vi "test-unscented-kalman-filter-1.vi"() -> (3 "Test good":bool)   [LabVIEW 2019]
uses:
  <vilib>/Analysis/Matrix/Datatypes/RealMatrix.ctl
  <vilib>/Rock Robotics/WPI/ThirdParty/JAS_Junk/TrajLib/TRAJ_STATE.ctl
  <vilib>/Rock Robotics/WPI/ThirdParty/JAS_Junk/TrajLib/POSE2D.ctl
  <vilib>/Rock Robotics/WPI/ThirdParty/JAS_Junk/TrajLib/TRANSLATION2D.ctl
  <vilib>/Rock Robotics/WPI/ThirdParty/JAS_Junk/TrajLib/ROTATION2D.ctl
  <vilib>/Rock Robotics/WPI/ThirdParty/JAS_Junk/TrajLib/MatrixHelper_CoerceSize.vi
  <vilib>/Rock Robotics/WPI/ThirdParty/JAS_Junk/TrajLib/Rotation_CreateAngle.vi
  <vilib>/Rock Robotics/WPI/ThirdParty/JAS_Junk/TrajLib/Translation_Create.vi
  <vilib>/Analysis/1siggen.llb/Gaussian White Noise.vi
  <vilib>/Analysis/Matrix/Numeric/Add/Add - RM,RM.vi
  <vilib>/Analysis/Matrix/Numeric/Subtract/Subtract - RM,RM.vi
  <vilib>/Analysis/7linalg.llb/Solve Linear Equations (multiple right hand).vi
  <vilib>/Rock Robotics/WPI/ThirdParty/JAS_Junk/TrajLib/CallbackHelp_MatrixPlus.vi
  <vilib>/Rock Robotics/WPI/ThirdParty/JAS_Junk/TrajLib/CallbackHelp_MatrixMinus.vi
  <vilib>/Rock Robotics/WPI/ThirdParty/JAS_Junk/TrajLib/Trajectory_Library.lvlib
  <vilib>/Analysis/Matrix/NI_Matrix.lvlib
  <vilib>/Analysis/NI_AALPro.lvlib
panel:
  out "Traj sample":T1={"TimeSeconds"=0.0, "Velocity"=0.0, "Acceleration"=0.0, "POSE"={"TRANSLATION"={"X"=0.0, "Y"=0.0}, "ROTATION"={"VALUE"=0.0, "COS"=1.0, "SIN"=0.0}}, "Curvature"=0.0} {"POSE"."ROTATION"."SIN" format="%13.4f"; "POSE"."ROTATION"."COS" format="%13.4f"; "POSE"."ROTATION"."VALUE" format="%13.4f"; "POSE"."TRANSLATION"."Y" format="%14.3f"; "POSE"."TRANSLATION"."X" format="%14.3f"}
  out "Error 14":bool
  out "xHat":T5
  out "OutputTRAJ_STATE":T1={"TimeSeconds"=0.0, "Velocity"=0.0, "Acceleration"=0.0, "POSE"={"TRANSLATION"={"X"=0.0, "Y"=0.0}, "ROTATION"={"VALUE"=0.0, "COS"=1.0, "SIN"=0.0}}, "Curvature"=0.0} {"POSE"."ROTATION"."SIN" format="%13.4f"; "POSE"."ROTATION"."COS" format="%13.4f"; "POSE"."ROTATION"."VALUE" format="%13.4f"; "POSE"."TRANSLATION"."Y" format="%14.3f"; "POSE"."TRANSLATION"."X" format="%14.3f"}
  out "Error 13":bool
  out "Sze Coerced":bool
  out "Error 12":errorcluster
  out "Return 2":T5
  out "Error 11":bool
  out "Error 10":bool
  out "Error 8":bool
  out "error":i32
  out "Solution Matrix":T5
  out "Get Dynam":T5
  out "Error 9":bool
  out "Size Coerced":bool
  out "TrueXHat":T5
  out "Error 3":bool
  out "Error 2":bool
  out "Error":bool
  out "r":T5
  out "SizeCoerced":bool
  out "X":T5
  out "Error 7":bool
  out "B":T5
  out "Y 2":T5
  out "Error 6":bool
  out "Error 5":bool
  out "Error 00":errorcluster
  # "assertEquals(finalPosition.poseMeters.getTranslation().getX(), observer.getXhat(0), 0.25);\n    assertEquals(finalPosition.poseMeters.getTranslation().getY(), observer.getXhat(1), 0.25);\n    assertEquals(finalPosition.poseMeters.getRotation().getRadians(), observer.getXhat(2), 1.0);\n    assertEquals(0.0, observer.getXhat(3), 1.0);\n    assertEquals(0.0, observer.getXhat(4), 1.0);"
  # "24.7"
  # "19.68"
  # "-.4372"
  # "0"
  # "0"
  # "Traj end\n          24.73, \n         19.68, \n          Degrees(5.846)"
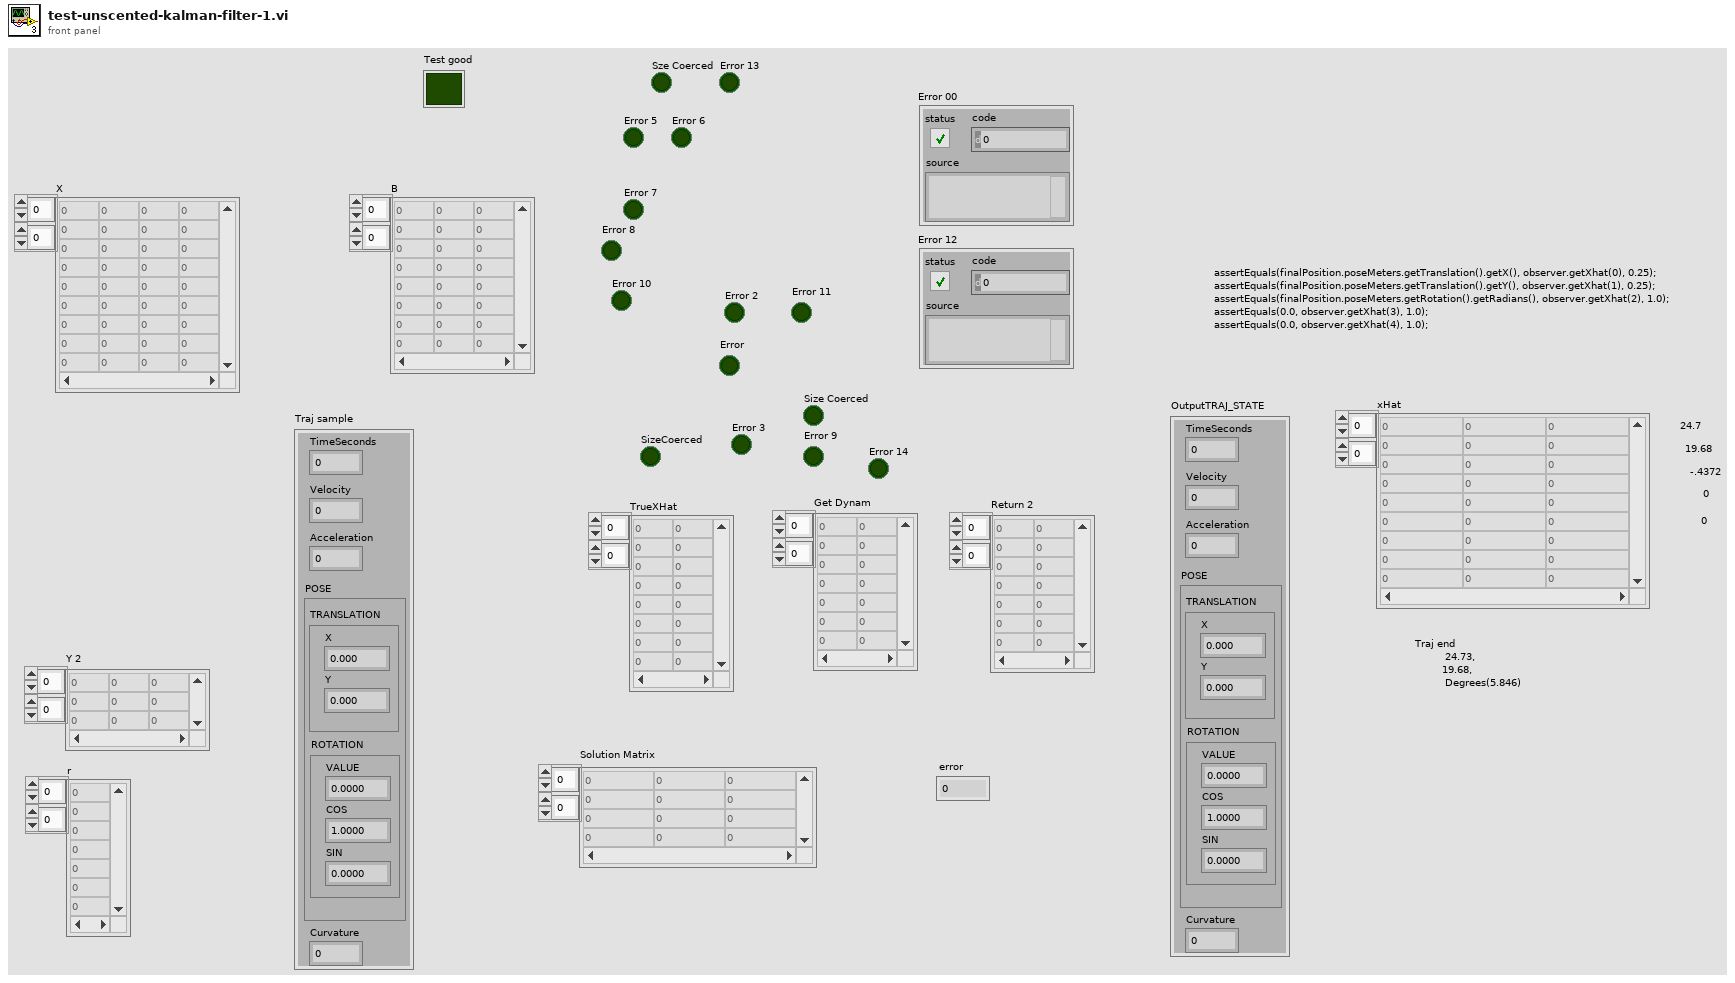
[diagram p1: front panel]
types:
  T1 = typedef "Trajectory_Library.lvlib/TRAJ_STATE.ctl" = cluster{"TimeSeconds":dbl, "Velocity":dbl, "Acceleration":dbl, "POSE":T2, "Curvature":dbl}
  T2 = typedef "Trajectory_Library.lvlib/POSE2D.ctl" = cluster{"TRANSLATION":T3, "ROTATION":T4}
  T3 = typedef "Trajectory_Library.lvlib/TRANSLATION2D.ctl" = cluster{"X":dbl, "Y":dbl}
  T4 = typedef "Trajectory_Library.lvlib/ROTATION2D.ctl" = cluster{"VALUE":dbl, "COS":dbl, "SIN":dbl}
  T5 = typedef "NI_Matrix.lvlib/RealMatrix.ctl" = dbl[][]
  T6 = typedef "Trajectory_Library.lvlib/TRAJ_CONFIG.ctl" = cluster{"MaxVelocity":dbl, "Max Acceleration":dbl, "StartVelocity":dbl, "End Velocity":dbl, "Reversed":bool, "DiffDrKineConstntDefined":bool, "CentAcellConstntDefined":bool, "DiffDrVoltConstntDefined":bool, "DIFF_DRIVE_KINE_CONSTRAINT":T7, "CENTRIPETAL_ACCEL_CONSTRAINT":T9, "SwerveDrKineConstntDefined":bool, "SWERVE_DRIVE_KINE_CONSTRAINT":T10, "DIFF_DRIVE_VOLTAGE_CONSTRAINT":T12, "MECANUM_DRIVE_KINE_CONSTRAINT":T14, "MecanumDrKineConstntDefined":bool}
  T7 = typedef "Trajectory_Library.lvlib/TRAJ_CONSTRAINT_DIIF_DRIVE_KINEMATICS.ctl" = cluster{"Max Speed (M/S)":dbl, "DIFF_DRIVE_KINEMATICS":T8, "Max Accel (M/S2)":dbl}
  T8 = typedef "Trajectory_Library.lvlib/DIFF_DRIVE_KINEMATICS.ctl" = cluster{"TrackWidth_Meters":dbl}
  T9 = typedef "Trajectory_Library.lvlib/TRAJ_CONSTRAINT_CENTRIPETAL_ACCEL.ctl" = cluster{"Max Cent Accel":dbl}
  T10 = typedef "Trajectory_Library.lvlib/TRAJ_CONSTRAINT_SWERVE_DRIVE_KINEMATICS.ctl" = cluster{"Max Speed (M/S)":dbl, "SwerveKinematics":T11}
  T11 = typedef "Trajectory_Library.lvlib/SWERVE_DRIVE_KINEMATICS.ctl" = cluster{"NumModules":i32, "InverseKinematics":T5, "ForwardKinematics":T5, "Modules":T3[], "PrevCoR":T3}
  T12 = typedef "Trajectory_Library.lvlib/TRAJ_CONSTRAINT_DIIF_DRIVE_VOLTAGE.ctl" = cluster{"Max Voltage":dbl, "DIFF_DRIVE_KINEMATICS":T8, "SIMPLE_MOTOR_FF":T13}
  T13 = typedef "Trajectory_Library.lvlib/SIMPLE_MOTOR_FF.ctl" = cluster{"Ks":dbl, "Kv":dbl, "Ka":dbl}
  T14 = typedef "Trajectory_Library.lvlib/TRAJ_CONSTRAINT_MECA_DRIVE_KINEMATICS.ctl" = cluster{"Max Speed (M/S)":dbl, "MECA_DRIVE_KINEMATICS":T15}
  T15 = typedef "Trajectory_Library.lvlib/MECA_DRIVE_KINEMATICS.ctl" = cluster{"FrontLeft":T3, "FrontRight":T3, "RearLeft":T3, "RearRight":T3, "InverseKinematics":T5, "ForwardKinematics":T5, "PrevCoR":T3}
  T16 = typedef "Trajectory_Library.lvlib/TRAJECTORY.ctl" = cluster{"TotalTImeSecs":dbl, "States":T1[]}
  T17 = typedef "Trajectory_Library.lvlib/UNSCENTED_KALMAN_FILTER.ctl" = cluster{"m_P":T5, "m_xHat":T5, "States":i32, "Outputs":i32, "m_ContR":T5, "m_ContQ":T5, "m_SigmasF":T5, "m_dT_Sec":dbl, "MERWE_SCALED_SIGMA_PTS":T18, "meanFuncX":T19, "meanFuncY":T19, "residualFuncX":T19, "residualFuncY":T19, "addFuncX":T19, "addFuncXExtra":variant, "residualFuncYExtra":variant, "residualFuncXExtra":variant, "MeanFuncYExtra":variant, "MeanFuncXExtra":variant, "Inputs":i32}
  T18 = typedef "Trajectory_Library.lvlib/MERWE_SCALED_SIGMA_PTS.ctl" = cluster{"m_Wm":T5, "States":i32, "Alpha":dbl, "m_Wc":T5, "Kappa":i32}
  T19 = typedef "Trajectory_Library.lvlib/CALLBACK_FUNC_TYPE.ctl" = refnum<vi>
  T20 = typedef "Trajectory_Library.lvlib/UNSCENTED_KALMAN_CORRECT_FUNC_GROUP.ctl" = cluster{"H_Func":T19, "meanFuncY":T19, "residualFuncY":T19, "residualFuncX":T19, "addFuncX":T19, "H_FuncExtra":variant, "MeanFuncYExtra":variant, "residualFuncYExtra":variant, "residualFuncXExtra":variant, "addFuncXExtra":variant}
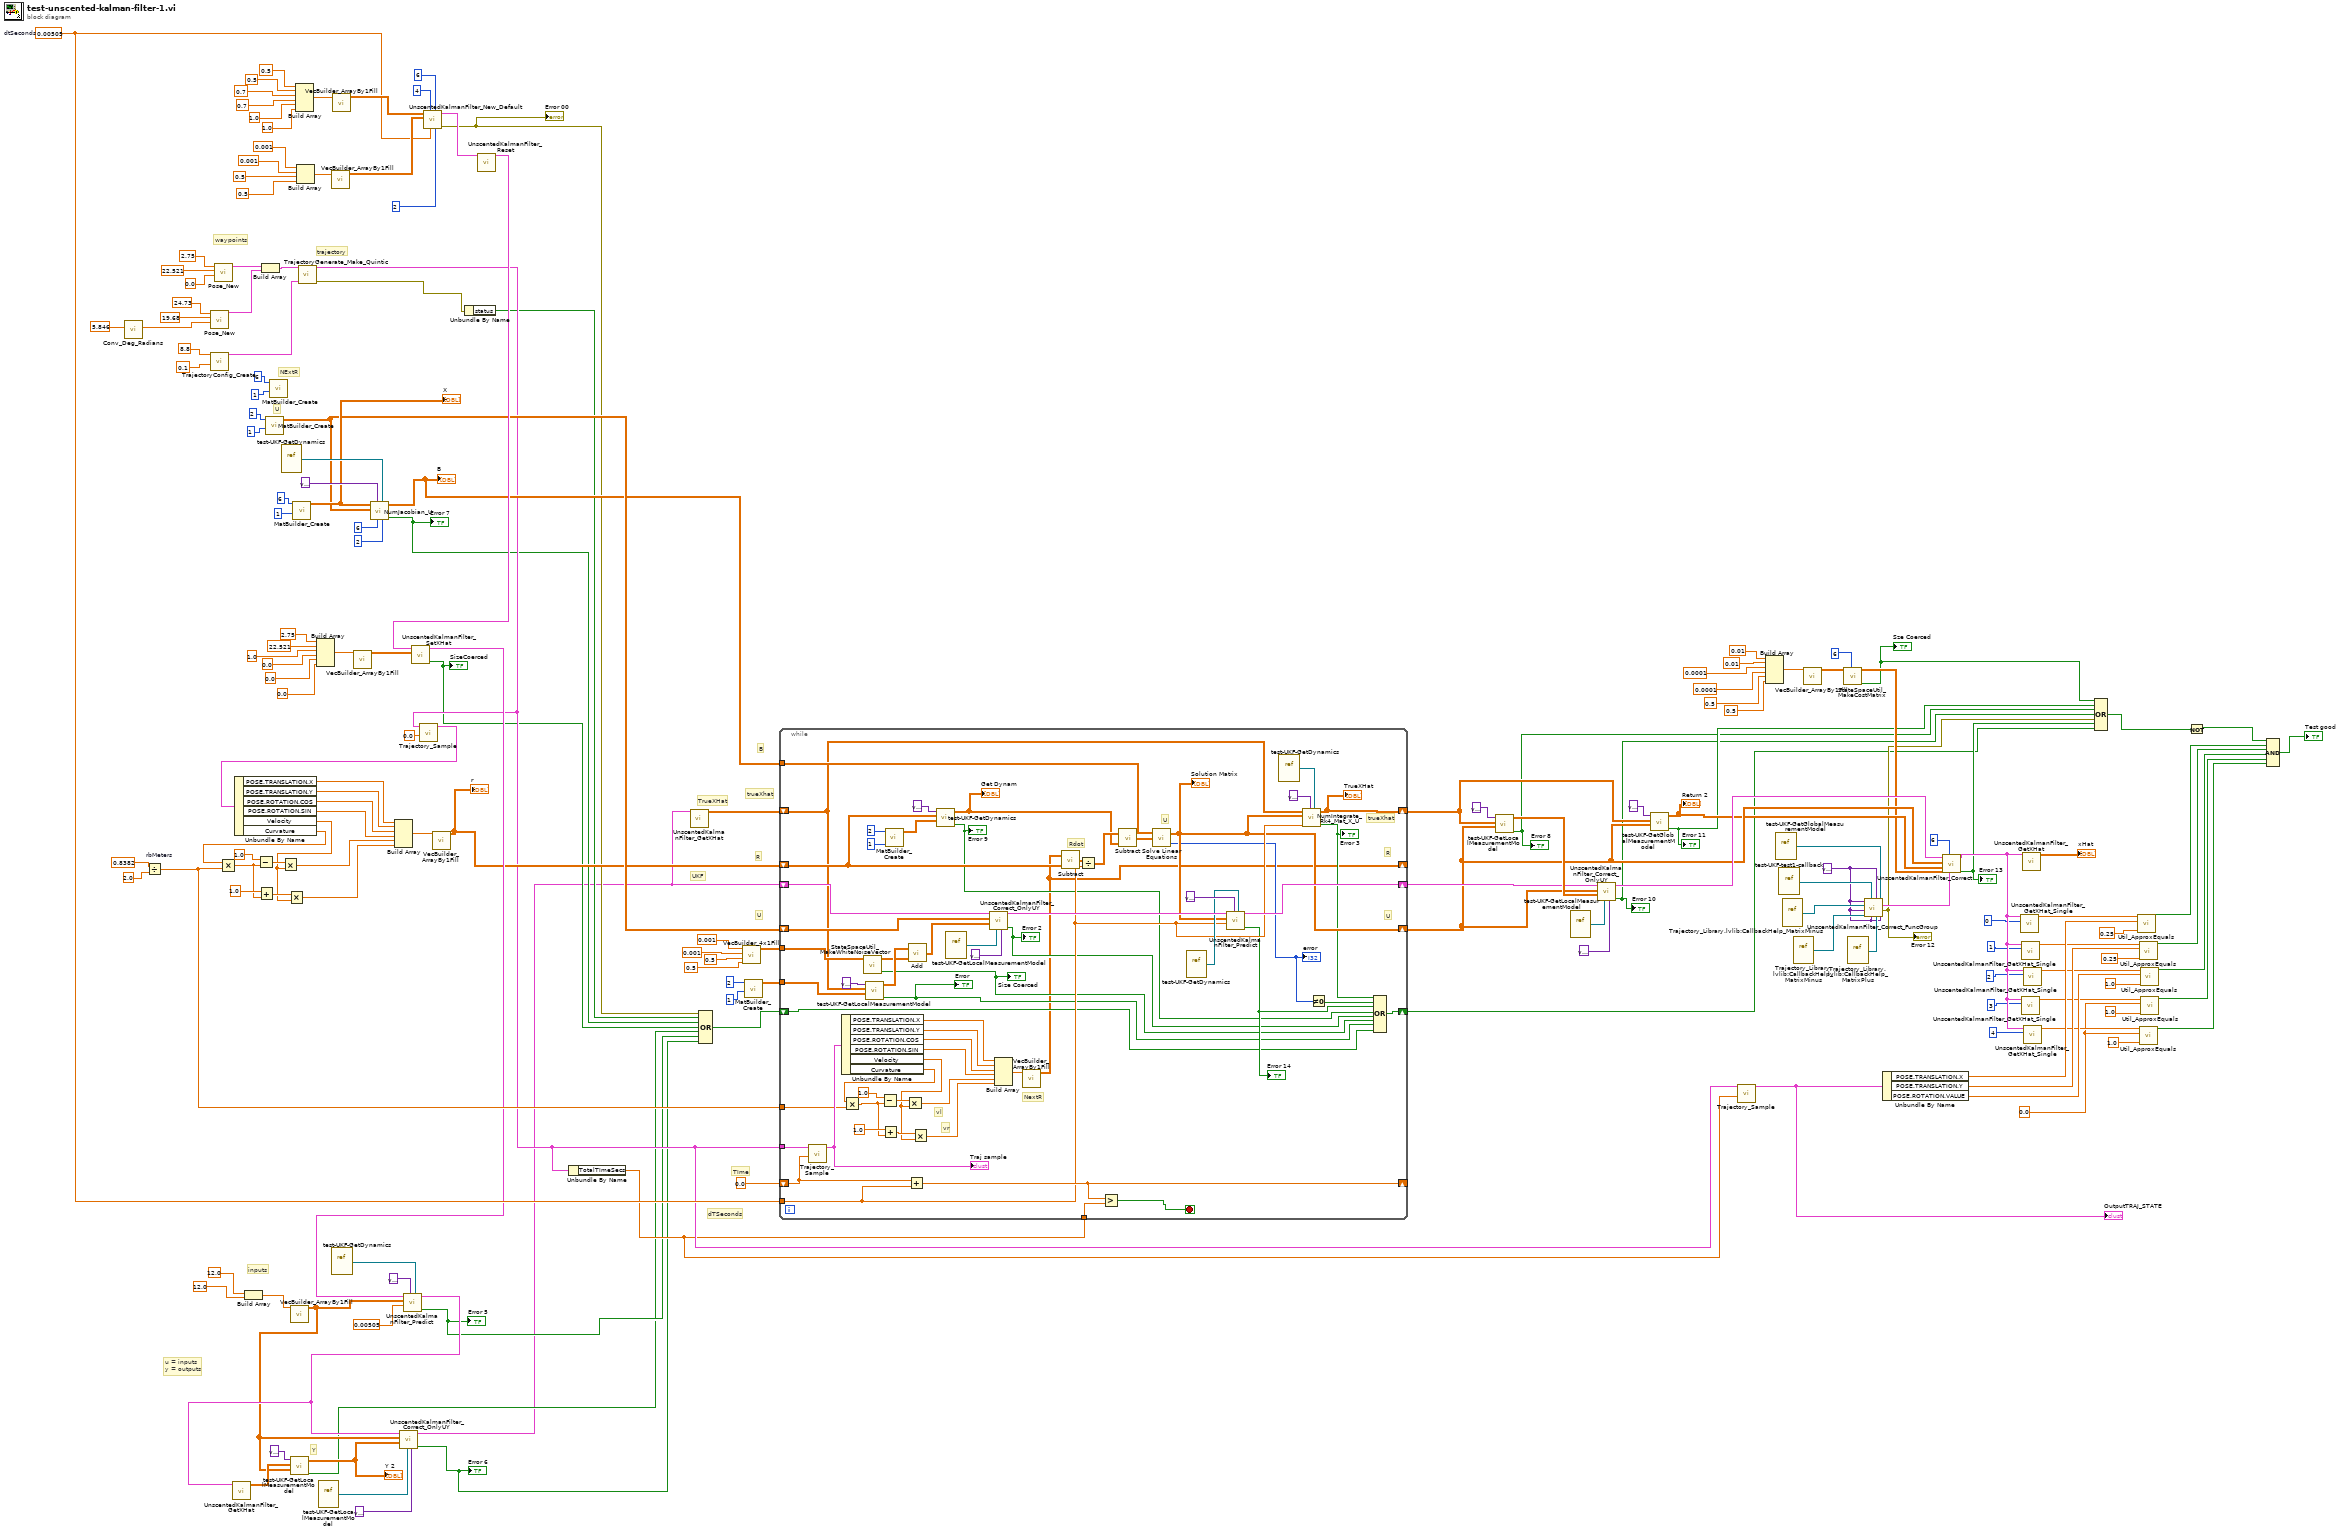
[diagram p0: block diagram]
diagram:
  w32 = 0.0 ("Value 2")
  w56 = variant ("H_FuncExtra")
  w93 = 0.00505  # dtSeconds
  # "UKF"
  # "B"
  # "trueXhat"
  # "dTSeconds"
  # "R"
  # "U"
  # "TrueXHat"
  # "TIme"
  # "U"
  # "NExtR"
  # "trajectory"
  # "waypoints"
  # "u = inputs\ny = outputs"
  # "inputs"
  # "Y"
  n1 = call <vilib>:"Conv_Deg_Radians.vi"("Degress"=5.846 ("Heading")) -> ("Radians"=w46:dbl)  [unwired: 10 in]
  n2 = Divide "rbMeters"(x=0.8382, y=2.0) -> (x/y=w92:dbl)
  n3 = call <vilib>:"Pose_New.vi"("Heading"=w46, "Y"=19.68, "X"=24.73) -> ("out POSe"=w135:T2)  [unwired: 8 in]
  n4 = call <vilib>:"TrajectoryConfig_Create.vi"("MaxAcceleration"=0.1, "MaxVelocity"=8.8) -> ("TRAJECTORY_CONFIG"=w131:T6)  [unwired: 9 in]
  n5 = call <vilib>:"Pose_New.vi"("Heading"=0.0, "Y"=22.521, "X"=2.75) -> ("out POSe"=w136:T2)  [unwired: 8 in]
  n6 = Build Array(12.0 ("element"), 12.0 ("element")) -> (w154:dbl[])
  n7 = Build Array(w136, w135) -> (w132:T2[])
  n8 = call <vilib>:"MatBuilder_Create.vi"("Columns"=1, "Rows"=2) -> ("output matrix"=w81:T5)  [unwired: 9 in]
  n9 = call <vilib>:"MatBuilder_Create.vi"("Columns"=1, "Rows"=6) -> ()  [unwired: 9 in, 1 out]
  n10 = vi-ref "test-UKF-GetDynamics.vi"() -> (w122:refnum<vi>)
  n11 = call <vilib>:"VecBuilder_ArrayBy1Fill.vi"("R Array"=w154) -> ("Output Vector"=w145:T5)  [unwired: 10 in]
  n12 = call <vilib>:"MatBuilder_Create.vi"("Columns"=1, "Rows"=6) -> ("output matrix"=w120:T5)  [unwired: 9 in]
  "X" <- w120
  n13 = Build Array(0.5 ("element"), 0.5 ("element"), 0.7 ("element"), 0.7 ("element"), 1.0 ("element"), 1.0 ("element")) -> (w172:dbl[])
  n14 = Build Array(0.001 ("element"), 0.001 ("element"), 0.5 ("element"), 0.5 ("element")) -> (w161:dbl[])
  n15 = call <vilib>:"TrajectoryGenerate_Make_Quintic.vi"("traj_config"=w131, "waypointPOSE"=w132) -> ("error out"=w10:errorcluster, "TRAJECTORY"=w50:T16)  [unwired: 8 in]
  n16 = Build Array(2.75 ("element"), 22.521 ("element"), 1.0 ("element"), 0.0 ("element"), 0.0 ("element"), 0.0 ("element")) -> (w112:dbl[])
  n17 = vi-ref "test-UKF-GetLocalMeasurementModel.vi"() -> (w149:refnum<vi>)
  n18 = call <vilib>:"VecBuilder_ArrayBy1Fill.vi"("R Array"=w161) -> ("Output Vector"=w160:T5)  [unwired: 10 in]
  n19 = vi-ref "test-UKF-GetDynamics.vi"() -> (w151:refnum<vi>)
  n20 = call <vilib>:"VecBuilder_ArrayBy1Fill.vi"("R Array"=w172) -> ("Output Vector"=w159:T5)  [unwired: 10 in]
  n21 = call <vilib>:"VecBuilder_ArrayBy1Fill.vi"("R Array"=w112) -> ("Output Vector"=w111:T5)  [unwired: 10 in]
  n22 = call <vilib>:"NumJacobian_U.vi"("Inputs"=2, "F_FUNC"=w122, "Rows"=6, "ExtraPassedData"=variant ("F_Func_ExtraData"), "U"=w81, "X"=w120) -> ("Error"=w11:bool, "Result"=w79:T5)  [unwired: 4 in]
  "B" <- w79
  "Error 7" <- w11
  n23 = call <vilib>:"Trajectory_Sample.vi"("Time"=0.0, "InputTRAJECTORY"=w50) -> ("OutputTRAJ_STATE"=w109:T1)  [unwired: 9 in]
  n24 = Unbundle By Name(w109) -> ("POSE.TRANSLATION.X"=w108:dbl, "POSE.TRANSLATION.Y"=w107:dbl, "POSE.ROTATION.COS"=w106:dbl, "POSE.ROTATION.SIN"=w105:dbl, "Velocity"=w98:dbl, "Curvature"=w104:dbl)
  n25 = Multiply(x=w104, y=w92) -> (x*y=w101:dbl)
  n26 = Subtract(x=1.0, y=w101) -> (x-y=w99:dbl)
  n27 = Add(x=1.0, y=w101) -> (x+y=w100:dbl)
  n28 = Multiply(x=w99, y=w98) -> (x*y=w97:dbl)
  n29 = Multiply(x=w100, y=w98) -> (x*y=w96:dbl)
  n30 = Build Array(w108, w107, w106, w105, w97, w96) -> (w95:dbl[])
  n31 = call <vilib>:"UnscentedKalmanFilter_New_Default.vi"("Inputs"=2, "States"=6, "dt_Seconds"=w93, "Outputs"=4, "MeasurementStdDevs"=w160, "StateStdDevs"=w159) -> ("Error"=w8:errorcluster, "UnscentedKalmanFiilter"=w157:T17)  [unwired: 4 in]
  "Error 00" <- w8
  n32 = call <vilib>:"VecBuilder_ArrayBy1Fill.vi"("R Array"=w95) -> ("Output Vector"=w80:T5)  [unwired: 10 in]
  "r" <- w80
  n33 = Unbundle By Name(w10) -> ("status"=w9:bool)
  n34 = call <vilib>:"UnscentedKalmanFilter_Reset.vi"("in UnscentedKalmanFiilter"=w157) -> ("out UnscentedKalmanFiilter"=w119:T17)  [unwired: 10 in]
  n35 = call <vilib>:"UnscentedKalmanFilter_SetXHat.vi"("xHat"=w111, "in UnscentedKalmanFiilter"=w119) -> ("SizeCoerced"=w13:bool, "out UnscentedKalmanFiilter"=w83:T17)  [unwired: 8 in]
  "SizeCoerced" <- w13
  n36 = call <vilib>:"UnscentedKalmanFilter_Predict.vi"("f_Func"=w151, "F_Func_ExtraData"=variant, "dT_Seconds"=0.00505, "U"=w145, "in UnscentedKalmanFiilter"=w83) -> ("Error"=w16:bool, "out UnscentedKalmanFiilter"=w148:T17)  [unwired: 5 in]
  "Error 5" <- w16
  n37 = call <vilib>:"UnscentedKalmanFilter_GetXHat.vi"("in UnscentedKalmanFiilter"=w148) -> ("xHat"=w146:T5)  [unwired: 10 in]
  n38 = call "test-UKF-GetLocalMeasurementModel.vi"("U"=w145, "X"=w146, "Variant"=variant) -> ("Error"=w14:bool, "Return"=w144:T5)  [unwired: 7 in]
  "Y 2" <- w144
  n39 = call <vilib>:"UnscentedKalmanFilter_Correct_OnlyUY.vi"("H_ExtraData"=variant ("F_Func_ExtraData"), "H_Func"=w149, "Y"=w144, "U"=w145, "in UnscentedKalmanFiilter"=w148) -> ("Error"=w15:bool, "out UnscentedKalmanFiilter"=w1:T17)  [unwired: 5 in]
  "Error 6" <- w15
  n40 = Unbundle By Name(w50) -> ("TotalTImeSecs"=w49:dbl)
  n41 = call <vilib>:"UnscentedKalmanFilter_GetXHat.vi"("in UnscentedKalmanFiilter"=w1) -> ("xHat"=w91:T5)  [unwired: 10 in]
  n42 = Compound Arithmetic op=OR(w8, w9, w11, w13, w14, w16, w15) -> (w12:bool)
  n43 = call <vilib>:"VecBuilder_4x1Fill.vi"("R3"=0.5, "R2"=0.5, "R1"=0.001, "R0"=0.001) -> ("output matrix"=w82:T5)  [unwired: 7 in]
  n44 = call <vilib>:"MatBuilder_Create.vi"("Columns"=1, "Rows"=2) -> ("output matrix"=w88:T5)  [unwired: 9 in]
  n45 = while {
    shift-right: [w235] -> _
    shift-left: 0.0 -> [w237]
    tunnel: w93 -> [w190]
    tunnel: w50 -> [w234]
    tunnel: w49 -> [w233]
    tunnel: w92 -> [w218]
    tunnel: w88 -> [w216]
    shift-right: [w197] -> w76
    shift-left: w1 -> [w215]
    tunnel: w82 -> [w214]
    shift-right: [w188] -> w53
    shift-left: w81 -> [w208]
    shift-right: [w176] -> _
    shift-left: w80 -> [w204]
    tunnel: w79 -> [w198]
    shift-right: [w189] -> w72
    shift-left: w91 -> [w191]
    shift-right: [w180] -> w7
    shift-left: w12 -> [w177]
    stop <- w236 stop-if-true
    # "vr"
    # "vl"
    # "Rdot"
    # "trueXhat"
    # "R"
    # "U"
    # "U"
    # "NextR"
    n46 = call <vilib>:"Trajectory_Sample.vi"("Time"=w237, "InputTRAJECTORY"=w234) -> ("OutputTRAJ_STATE"=w219:T1)  [unwired: 9 in]
    "Traj sample" <- w219
    n47 = Unbundle By Name(w219) -> ("POSE.TRANSLATION.X"=w232:dbl, "POSE.TRANSLATION.Y"=w231:dbl, "POSE.ROTATION.COS"=w230:dbl, "POSE.ROTATION.SIN"=w229:dbl, "Velocity"=w222:dbl, "Curvature"=w228:dbl)
    n48 = Multiply(x=w228, y=w218) -> (x*y=w225:dbl)
    n49 = call <vilib>:"StateSpaceUtil_MakeWhiteNoiseVector.vi"("StdDevs"=w214) -> ("Size Coerced"=w179:bool, "WhiteNoise"=w211:T5)  [unwired: 9 in]
    "Size Coerced" <- w179
    n50 = call "test-UKF-GetLocalMeasurementModel.vi"("U"=w216, "X"=w191, "Variant"=variant) -> ("Error"=w178:bool, "Return"=w212:T5)  [unwired: 7 in]
    "Error" <- w178
    n51 = Subtract(x=1.0, y=w225) -> (x-y=w223:dbl)
    n52 = Add(x=1.0, y=w225) -> (x+y=w224:dbl)
    n53 = call <vilib>:"MatBuilder_Create.vi"("Columns"=1, "Rows"=2) -> ("output matrix"=w200:T5)  [unwired: 9 in]
    n54 = Multiply(x=w223, y=w222) -> (x*y=w221:dbl)
    n55 = Add(x=w237, y=w190) -> (x+y=w235:dbl)
    n56 = call-poly <vilib>:"Add.vi"("Real Matrix B"=w211, "Real Matrix A"=w212) -> ("A + B"=w213:T5)
    n57 = Multiply(x=w224, y=w222) -> (x*y=w220:dbl)
    n58 = call "test-UKF-GetDynamics.vi"("U"=w200, "X"=w204, "Variant"=variant) -> ("Error"=w182:bool, "Return"=w183:T5)  [unwired: 7 in]
    "Error 9" <- w182
    "Get Dynam" <- w183
    n59 = vi-ref "test-UKF-GetLocalMeasurementModel.vi"() -> (w210:refnum<vi>)
    n60 = call <vilib>:"UnscentedKalmanFilter_Correct_OnlyUY.vi"("H_ExtraData"=variant, "H_Func"=w210, "Y"=w213, "U"=w208, "in UnscentedKalmanFiilter"=w215) -> ("Error"=w181:bool, "out UnscentedKalmanFiilter"=w196:T17)  [unwired: 5 in]
    "Error 2" <- w181
    n61 = Build Array(w232, w231, w230, w229, w221, w220) -> (w207:dbl[])
    n62 = call <vilib>:"VecBuilder_ArrayBy1Fill.vi"("R Array"=w207) -> ("Output Vector"=w176:T5)  [unwired: 10 in]
    n63 = call-poly <vilib>:"Subtract.vi"("Real Matrix B"=w204, "Real Matrix A"=w176) -> ("A - B"=w206:T5)
    n64 = Divide(x=w206, y=w190) -> (x/y=w205:T5)
    n65 = Greater?(x=w235, y=w233) -> (0:w236:bool)
    n66 = call-poly <vilib>:"Subtract.vi"("Real Matrix B"=w183, "Real Matrix A"=w205) -> ("A - B"=w199:T5)
    n67 = call-poly <vilib>:"Solve Linear Equations.vi"("Known Matrix"=w199, "Input Matrix"=w198) -> ("error"=w185:i32, "Solution Matrix"=w188:T5)  [unwired: 1 in]
    "Solution Matrix" <- w188
    "error" <- w185
    n68 = vi-ref "test-UKF-GetDynamics.vi"() -> (w194:refnum<vi>)
    n69 = call <vilib>:"UnscentedKalmanFilter_Predict.vi"("f_Func"=w194, "F_Func_ExtraData"=variant, "dT_Seconds"=w190, "U"=w188, "in UnscentedKalmanFiilter"=w196) -> ("Error"=w184:bool, "out UnscentedKalmanFiilter"=w197:T17)  [unwired: 5 in]
    "Error 14" <- w184
    n70 = vi-ref "test-UKF-GetDynamics.vi"() -> (w192:refnum<vi>)
    n71 = call <vilib>:"NumIntegrate_Rk4_Mat_X_U.vi"("Func_X_U_Extra"=w192, "PassedData"=variant, "dT_Seconds"=w190, "U"=w188, "X"=w191) -> ("Error"=w187:bool, "OUTPUT"=w189:T5)  [unwired: 5 in]
    "Error 3" <- w187
    "TrueXHat" <- w189
    n72 = Not Equal To 0?(x=w185) -> (x != 0?=w186:bool)
    n73 = Compound Arithmetic op=OR(w187, w186, w184, w182, w181, w179, w178, w177) -> (w180:bool)
  }
  n74 = call "test-UKF-GetLocalMeasurementModel.vi"("U"=w53, "X"=w72, "Variant"=variant) -> ("Error"=w27:bool, "Return"=w77:T5)  [unwired: 7 in]
  "Error 8" <- w27
  n75 = vi-ref "test-UKF-GetLocalMeasurementModel.vi"() -> (w75:refnum<vi>)
  n76 = call <vilib>:"UnscentedKalmanFilter_Correct_OnlyUY.vi"("H_ExtraData"=variant, "H_Func"=w75, "Y"=w77, "U"=w53, "in UnscentedKalmanFiilter"=w76) -> ("Error"=w26:bool, "out UnscentedKalmanFiilter"=w55:T17)  [unwired: 5 in]
  "Error 10" <- w26
  n77 = call "test-UKF-GetGlobalMeasurementModel.vi"("U"=w53, "X"=w72, "Variant"=variant) -> ("Error"=w28:bool, "Return"=w52:T5)  [unwired: 7 in]
  "Error 11" <- w28
  "Return 2" <- w52
  n78 = call <vilib>:"Trajectory_Sample.vi"("Time"=w49, "InputTRAJECTORY"=w50) -> ("OutputTRAJ_STATE"=w45:T1)  [unwired: 9 in]
  "OutputTRAJ_STATE" <- w45
  n79 = Build Array(0.01 ("element"), 0.01 ("element"), 0.0001 ("element"), 0.0001 ("element"), 0.5 ("element"), 0.5 ("element")) -> (w63:dbl[])
  n80 = vi-ref "test-UKF-GetGlobalMeasurementModel.vi"() -> (w57:refnum<vi>)
  n81 = vi-ref "test-UKF-test1-callback.vi"() -> (w58:refnum<vi>)
  n82 = vi-ref "Trajectory_Library.lvlib:CallbackHelp_MatrixMinus.vi"() -> (w59:refnum<vi>)
  n83 = vi-ref "Trajectory_Library.lvlib:CallbackHelp_MatrixMinus.vi"() -> (w60:refnum<vi>)
  n84 = call <vilib>:"VecBuilder_ArrayBy1Fill.vi"("R Array"=w63) -> ("Output Vector"=w64:T5)  [unwired: 10 in]
  n85 = call <vilib>:"StateSpaceUtil_MakeCostMatrix.vi"("States"=6, "Costs"=w64) -> ("Sze Coerced"=w29:bool, "Costs Matrix"=w51:T5)  [unwired: 8 in]
  "Sze Coerced" <- w29
  n86 = vi-ref "Trajectory_Library.lvlib:CallbackHelp_MatrixPlus.vi"() -> (w61:refnum<vi>)
  n87 = call <vilib>:"UnscentedKalmanFilter_Correct_FuncGroup.vi"("addFuncXExtra"=w56, "H_Func"=w57, "AddFuncX"=w61, "H_FuncExtra"=w56, "residualFuncXExtra"=w56, "MeanFuncY"=w58, "ResidualFuncX"=w60, "residualFuncYExtra"=w56, "ResidualFuncY"=w59, "MeanFuncYExtra"=w56) -> ("Error"=w25:errorcluster, "UNSCENTED_KALMAN_CORRECT_FUNC_GROUP"=w62:T20)
  "Error 12" <- w25
  n88 = Unbundle By Name(w45) -> ("POSE.TRANSLATION.X"=w42:dbl, "POSE.TRANSLATION.Y"=w39:dbl, "POSE.ROTATION.VALUE"=w36:dbl)
  n89 = call <vilib>:"UnscentedKalmanFilter_Correct.vi"("UNSCENTED_KALMAN_CORRECT_FUNC_GROUP"=w62, "Rows"=6, "R"=w51, "Y"=w52, "U"=w53, "in UnscentedKalmanFiilter"=w55) -> ("Error"=w24:bool, "out UnscentedKalmanFiilter"=w44:T17)  [unwired: 4 in]
  "Error 13" <- w24
  n90 = call <vilib>:"UnscentedKalmanFilter_GetXHat_Single.vi"("Row"=0, "in UnscentedKalmanFiilter"=w44) -> ("xHat Value"=w43:dbl)  [unwired: 9 in]
  n91 = call <vilib>:"UnscentedKalmanFilter_GetXHat_Single.vi"("Row"=1, "in UnscentedKalmanFiilter"=w44) -> ("xHat Value"=w40:dbl)  [unwired: 9 in]
  n92 = call <vilib>:"UnscentedKalmanFilter_GetXHat_Single.vi"("Row"=3, "in UnscentedKalmanFiilter"=w44) -> ("xHat Value"=w34:dbl)  [unwired: 9 in]
  n93 = call <vilib>:"UnscentedKalmanFilter_GetXHat.vi"("in UnscentedKalmanFiilter"=w44) -> ("xHat"=→"xHat":T5)  [unwired: 10 in]
  n94 = call <vilib>:"UnscentedKalmanFilter_GetXHat_Single.vi"("Row"=2, "in UnscentedKalmanFiilter"=w44) -> ("xHat Value"=w37:dbl)  [unwired: 9 in]
  n95 = call <vilib>:"UnscentedKalmanFilter_GetXHat_Single.vi"("Row"=4, "in UnscentedKalmanFiilter"=w44) -> ("xHat Value"=w33:dbl)  [unwired: 9 in]
  n96 = Compound Arithmetic op=OR(w29, w28, w27, w26, w25, w24, w7) -> (w18:bool)
  n97 = call <vilib>:"Util_ApproxEquals.vi"("Tolerance"=0.25, "Value 2"=w42, "Value 1"=w43) -> ("ApproxEquals"=w6:bool)  [unwired: 8 in]
  n98 = call <vilib>:"Util_ApproxEquals.vi"("Tolerance"=0.25, "Value 2"=w39, "Value 1"=w40) -> ("ApproxEquals"=w5:bool)  [unwired: 8 in]
  n99 = call <vilib>:"Util_ApproxEquals.vi"("Tolerance"=1.0, "Value 2"=w32, "Value 1"=w33) -> ("ApproxEquals"=w2:bool)  [unwired: 8 in]
  n100 = call <vilib>:"Util_ApproxEquals.vi"("Tolerance"=1.0, "Value 2"=w36, "Value 1"=w37) -> ("ApproxEquals"=w4:bool)  [unwired: 8 in]
  n101 = call <vilib>:"Util_ApproxEquals.vi"("Tolerance"=1.0, "Value 2"=w32, "Value 1"=w34) -> ("ApproxEquals"=w3:bool)  [unwired: 8 in]
  n102 = Not(x=w18) -> (.not. x?=w17:bool)
  n103 = Compound Arithmetic op=AND(w17, w6, w5, w4, w3, w2) -> (→"Test good":bool)
